vi "Set Plugin Thread Settings.vi"(8 "error in (no error)":errorcluster, 9 "custom settings":T1, 10 "plugin thread index":i32, 11 "plugin in":T2={"name"="Plugin", "components"=[], "cycle timing"={"priority"=10000, "decimation"=1, "offset"=0}, "threads"=[], "transfer groups"=[], "settings"=[]} {"transfer groups"."transfers"."channels"."string offset" format="%d bytes"}) -> (0 "error out":errorcluster, 3 "plugin out":T2={"name"="Plugin", "components"=[], "cycle timing"={"priority"=10000, "decimation"=1, "offset"=0}, "threads"=[], "transfer groups"=[], "settings"=[]} {"transfer groups"."transfers"."channels"."string offset" format="%d bytes"})   [LabVIEW 2017, in "DSF Core.lvlib" / "Configuration Session.lvclass"]
doc: "Determines whether a configuration data dsf refnum is valid."
uses:
  Configuration Session.lvclass
  Typedefs/DSF Engine Plugin Configuration.ctl
  Typedefs/DSF Timing Info.ctl
  Typedefs/DSF Engine Plugin Thread Configuration.ctl
  Typedefs/DSF Settings Info.ctl
  Typedefs/DSF Engine Transfer Group Configuration.ctl
  Typedefs/DSF Direction.ctl
  Typedefs/DSF Engine Transfer Configuration.ctl
  Typedefs/DSF Byte Order.ctl
  Typedefs/DSF Engine Channel Configuration.ctl
  Typedefs/DSF Data Type.ctl
  Typedefs/DSF Timeout Behavior.ctl
  DSF Core.lvlib
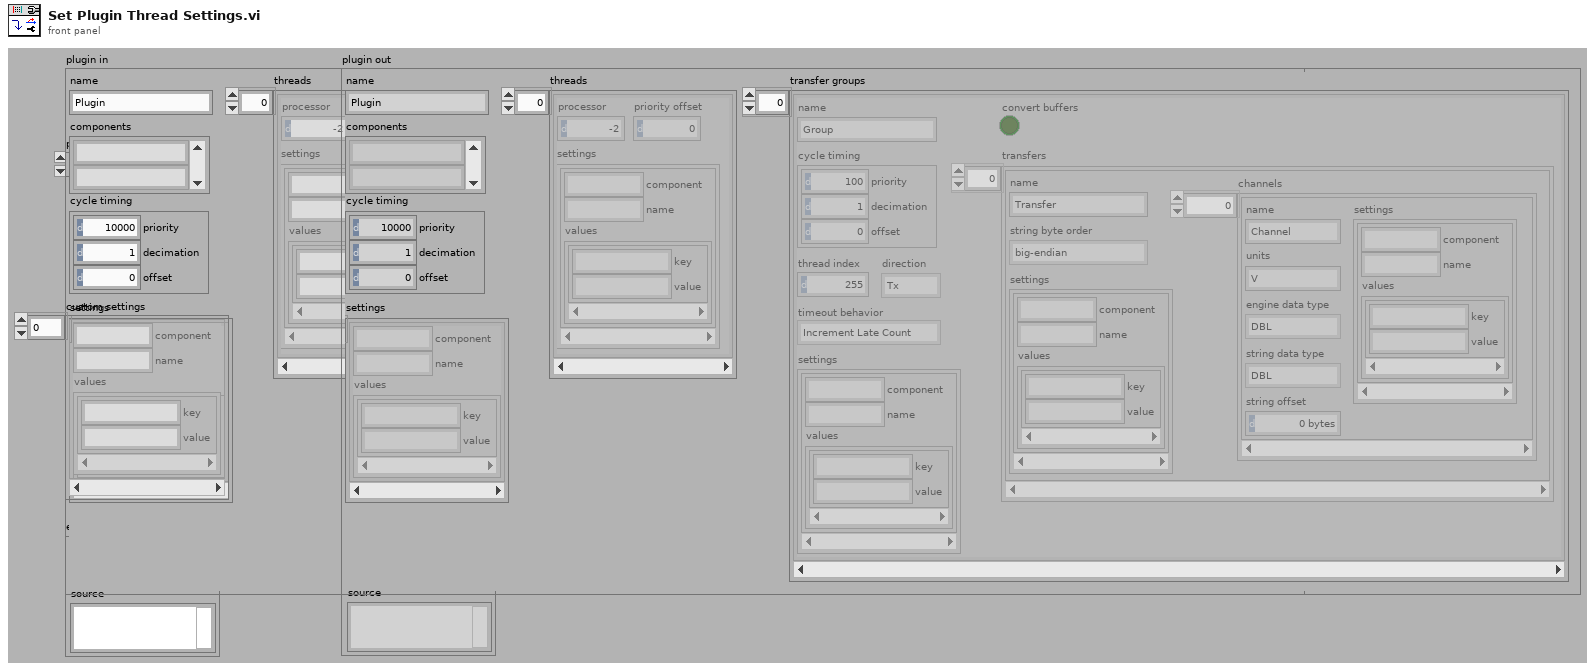
[diagram p1: front panel]
types:
  T1 = typedef "DSF Core.lvlib/DSF Settings Info.ctl" = cluster{"component":string, "name":string, "values":cluster{"key":string, "value":string}[]}[]
  T2 = typedef "DSF Core.lvlib/DSF Engine Plugin Configuration.ctl" = cluster{"name":string, "components":string[], "cycle timing":T3, "threads":T4[], "transfer groups":T5[], "settings":T1}
  T3 = typedef "DSF Core.lvlib/DSF Timing Info.ctl" = cluster{"priority":u64, "decimation":u64, "offset":u64}
  T4 = typedef "DSF Core.lvlib/DSF Engine Plugin Thread Configuration.ctl" = cluster{"processor":i32, "priority offset":i16, "settings":T1}
  T5 = typedef "DSF Core.lvlib/DSF Engine Transfer Group Configuration.ctl" = cluster{"name":string, "direction":T6, "cycle timing":T3, "thread index":u8, "settings":T1, "transfers":T7[], "timeout behavior":T11, "convert buffers":bool}
  T6 = typedef "DSF Core.lvlib/DSF Direction.ctl" = enum8{"Tx", "Rx"}
  T7 = typedef "DSF Core.lvlib/DSF Engine Transfer Configuration.ctl" = cluster{"name":string, "string byte order":T8, "settings":T1, "channels":T9[]}
  T8 = typedef "DSF Core.lvlib/DSF Byte Order.ctl" = enum8{"big-endian", "little-endian"}
  T9 = typedef "DSF Core.lvlib/DSF Engine Channel Configuration.ctl" = cluster{"string offset":u64, "name":string, "units":string, "engine data type":T10, "string data type":T10, "settings":T1}
  T10 = typedef "DSF Core.lvlib/DSF Data Type.ctl" = enum8{"Bool", "SGL", "DBL", "I8", "I16", "I32", "I64", "U8", "U16", "U32", "U64"}
  T11 = typedef "DSF Core.lvlib/DSF Timeout Behavior.ctl" = enum8{"Increment Late Count", "Throw Error"}
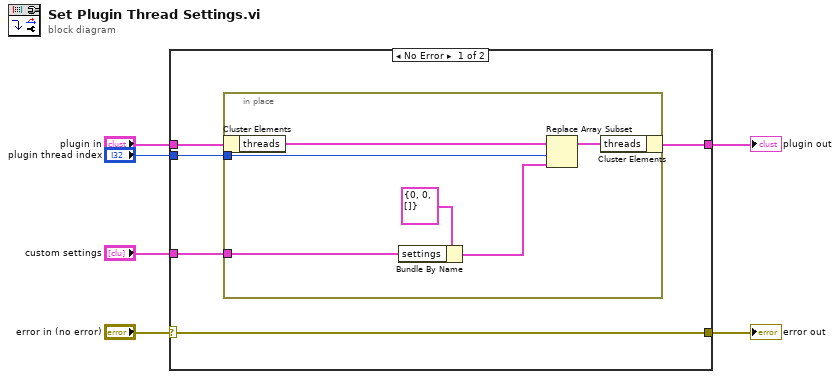
[diagram p0: block diagram]
diagram:
  n1 = case shown="No Error" "error in (no error)" {
    selector: "error in (no error)" -> [w9 w19]
    tunnel: [w9 w19] -> w6
    tunnel: "plugin in" -> [w11 w18]
    tunnel: [w10 w18] -> w3
    tunnel: "plugin thread index" -> [w8 _]
    tunnel: "custom settings" -> [w7 _]
    frame No Error {
      n2 = in-place {
        in-place-border: w8 -> [w13]
        in-place-border: w7 -> [w12]
        n3 = in-place-cluster #1(w11) -> ("threads"=w16:T4[])
        n4 = Bundle By Name(cluster=T4 {"processor"=0, "priority offset"=0, "settings"=[]} ("Plugin Thread Configuration"), "settings"=w12) -> (w14:T4)
        n5 = Replace Array Subset(array=w16, new element=w14, index=w13) -> (w15:T4[])
        n6 = in-place-cluster #1("threads"=w15) -> (w10:T2)
      }
    }
    frame Error {
    }
  }
  "error out" <- w6
  "plugin out" <- w3
